vi "Create.vi"(6 "advanced":T1, 8 "error in (no error)":errorcluster, 11 "service name":string) -> (0 "error out":errorcluster, 3 "service out":refnum<class "IcmMessageService.lvclass">)   [LabVIEW 2017, in "IcmMessageService.lvclass"]
doc: "Creates an NI InsightCM Server message bus session."
uses:
  <vilib>/addons/InsightCM/MessageBus/MessageService/IcmMessageService.lvclass
  <vilib>/addons/InsightCM/MessageBus/MessageService/controls/ServiceAdvancedConfig.ctl
  <vilib>/addons/InsightCM/MessageBus/MessageService/controls/MessageServiceData.ctl
  C:/Program Files (x86)/National Instruments/LabVIEW 2017/vi.lib/addons/InsightCM/Binaries/LabviewMessageAdapter.dll
  Binaries/LabviewMessageAdapter.dll
  <vilib>/addons/InsightCM/MessageBus/MessageService/IcmMessageService.lvclass/IcmMessageService.ctl
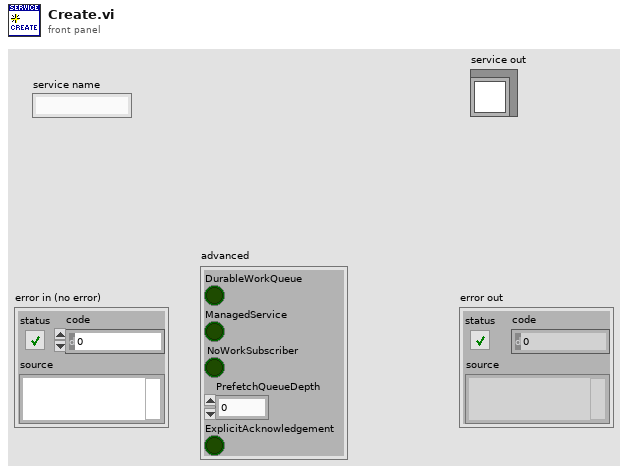
[diagram p1: front panel]
types:
  T1 = typedef "ServiceAdvancedConfig.ctl" = cluster{"DurableWorkQueue":bool, "ManagedService":bool, "NoWorkSubscriber":bool, "PrefetchQueueDepth":u16, "ExplicitAcknowledgement":bool}
  T2 = typedef "MessageServiceData.ctl" = cluster{"Service":refnum<k24>}
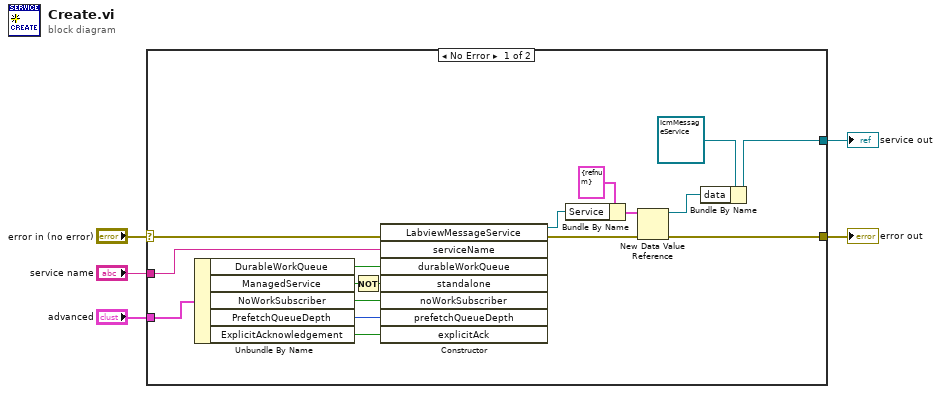
[diagram p0: block diagram]
diagram:
  n1 = case shown="No Error" "error in (no error)" {
    selector: "error in (no error)" -> [w14 w23]
    tunnel: [w13 w23] -> w4
    tunnel: [w22 _] -> w3
    tunnel: "service name" -> [w17 _]
    tunnel: "advanced" -> [w7 _]
    frame No Error {
      n2 = Unbundle By Name(w7) -> ("DurableWorkQueue"=w12:bool, "ManagedService"=w11:bool, "NoWorkSubscriber"=w10:bool, "PrefetchQueueDepth"=w9:u16, "ExplicitAcknowledgement"=w8:bool)
      n3 = Not(x=w11) -> (.not. x?=w6:bool)
      n4 = constructor class="LabviewMessageService"(error in=w14, "serviceName"=w17, "durableWorkQueue"=w12, "standalone"=w6, "noWorkSubscriber"=w10, "prefetchQueueDepth"=w9, "explicitAck"=w8) -> (reference out=w18:refnum<k24>, error out=w15:errorcluster)  [unwired: 2 in, 7 out]
      n5 = Bundle By Name(cluster=T2 {"Service"=refnum} ("MessageService"), "Service"=w18) -> (w19:T2)
      n6 = New Data Value Reference(data value=w19, error in=w15) -> (data value reference=w21:refnum<data-value>, error out=w13:errorcluster)
      n7 = Bundle By Name(cluster=refnum<class "IcmMessageService.lvclass"> refnum ("IcmMessageService in"), "data"=w21) -> (w22:refnum<class "IcmMessageService.lvclass">)
    }
    frame Error {
    }
  }
  "error out" <- w4
  "service out" <- w3
